vi "Read value.vi"(8 "Error In":errorcluster, 11 "obj in":refnum<class "TranscriptorBasicObject.lvclass">) -> (0 "Error Out":errorcluster, 2 "value":string, 3 "obj out":refnum<class "TranscriptorBasicObject.lvclass">)   [LabVIEW 2014, in "TranscriptorBasicObject.lvclass"]
uses:
  TranscriptorBasicObject.lvclass
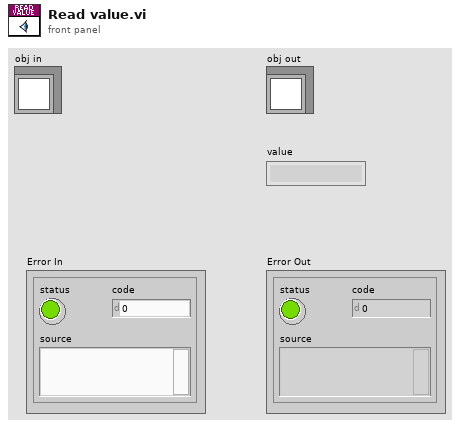
[diagram p1: front panel]
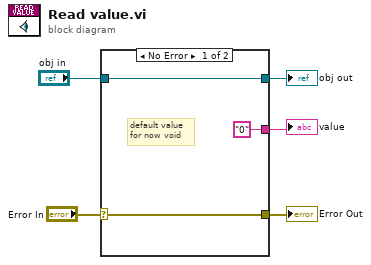
[diagram p0: block diagram]
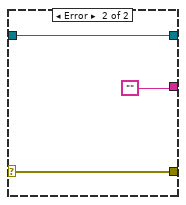
[diagram p2: hidden frame]
diagram:
  n1 = case shown="No Error" "Error In" {
    selector: "Error In" -> [w8 w10]
    tunnel: [w8 w10] -> w5
    tunnel: "obj in" -> [w7 w11]
    tunnel: [w7 w11] -> w2
    tunnel: ["0" ""] -> w1
    frame No Error {
      # "default value\nfor now void"
    }
    frame Error {
    }
  }
  "Error Out" <- w5
  "obj out" <- w2
  "value" <- w1
